vi "Msg.vi"(7 "Actor in":refnum<class "Actor.lvclass">, 11 "Actor Last Ack Msg Strategy in":refnum<class "Actor Last Ack Msg Strategy.lvclass">) -> (0 "error out":errorcluster, 5 "Actor out":refnum<class "Actor.lvclass">)   [LabVIEW 2021, in "Actor Last Ack.lvlib" / "Actor Last Ack Msg Strategy.lvclass"]
uses:
  Actor Last Ack Msg Strategy.lvclass
  LVCAM/Actor/Actor.lvclass
  Actor Last Ack/Actor Last Ack.lvclass
  26d28521-7f61-4032-a412-881153c4d1f0.vi
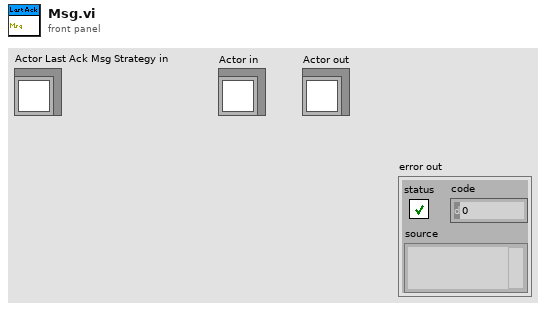
[diagram p1: front panel]
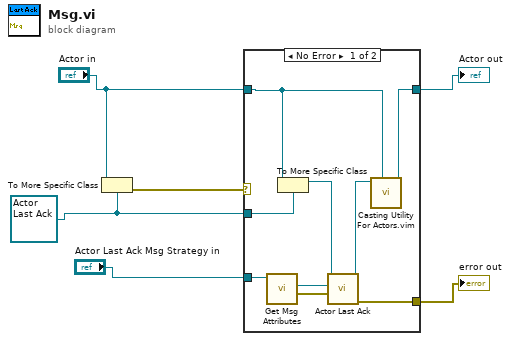
[diagram p0: block diagram]
diagram:
  w1 = refnum<class "Actor Last Ack.lvclass"> refnum ("Last Ack.lvlib:Last Ack.lvclass")
  n1 = To More Specific Class(target class=w1, reference="Actor in") -> (error out=w6:errorcluster)  [unwired: 1 in, 1 out]
  n2 = case shown="No Error" w6 {
    selector: w6 -> [_ w17]
    tunnel: [w7 w17] -> w5
    tunnel: [w14 w16] -> w4
    tunnel: "Actor in" -> [w13 w16]
    tunnel: w1 -> [w15 _]
    tunnel: "Actor Last Ack Msg Strategy in" -> [w12 _]
    frame No Error {
      n3 = call "Get Msg Attributes.vi"("Actor Last Ack Msg Strategy in"=w12) -> ("Nested Error"=w8:errorcluster, "Nested Actor"=w9:refnum<class "Actor.lvclass">)  [unwired: 9 in]
      n4 = To More Specific Class(target class=w15, reference=w13) -> (specific class reference=w10:refnum<class "Actor Last Ack.lvclass">)  [unwired: 1 in, 1 out]
      n5 = call-dynamic "Actor Last Ack.vi"("Nested Error"=w8, "Nested Actor"=w9, "Actor Last Ack in"=w10) -> ("error out"=w7:errorcluster, "Actor Last Ack out"=w11:refnum<class "Actor Last Ack.lvclass">)  [unwired: 7 in]
      n6 = call "Casting Utility For Actors.vim"("type"=w13, "Actor in"=w11) -> ("Actor out"=w14:refnum<class "Actor.lvclass">)  [unwired: 8 in, 1 out]
    }
    frame Error {
    }
  }
  "error out" <- w5
  "Actor out" <- w4
